vi "Joystick Controls.vi"() -> (3 "Input Cluster":T1)   [LabVIEW 2015]
uses:
  Joytsick/Joytstick Controls Type.ctl
  Global Vars.vi
  <vilib>/Rock Robotics/WPI/Utilities/WPI_GetSetVariantRefNum.vi
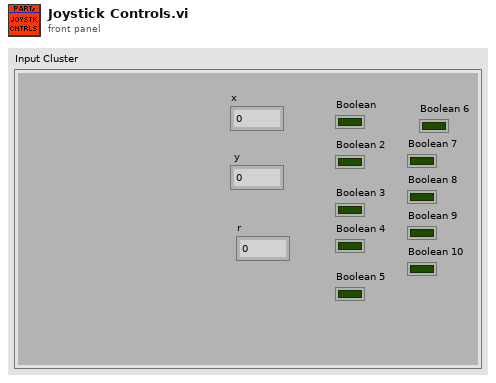
[diagram p1: front panel]
types:
  T1 = typedef "Joytstick Controls Type.ctl" = cluster{"x":dbl, " y":dbl, "r":dbl, "Boolean":bool, "Boolean 2":bool, "Boolean 3":bool, "Boolean 4":bool, "Boolean 5":bool, "Boolean 6":bool, "Boolean 7":bool, "Boolean 8":bool, "Boolean 9":bool, "Boolean 10":bool}
  T2 = typedef "WPI_JoystickDevRef.ctl" = cluster{"Device":T3}
  T3 = typedef "WPI_JoystickDeviceEnum.ctl" = enum16{"USB 0", "USB 1", "USB 2", "USB 3", "USB 4", "USB 5"}
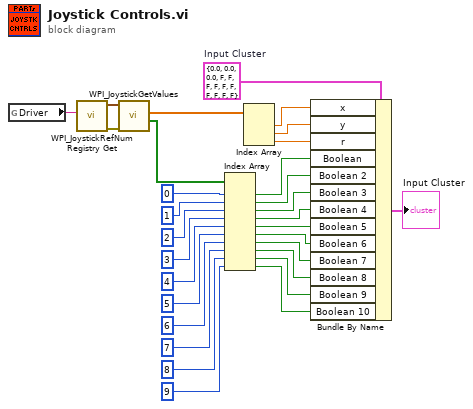
[diagram p0: block diagram]
diagram:
  w18 = T1 {"x"=0.0, " y"=0.0, "r"=0.0, "Boolean"=FALSE, "Boolean 2"=FALSE, "Boolean 3"=FALSE, "Boolean 4"=FALSE, "Boolean 5"=FALSE, "Boolean 6"=FALSE, "Boolean 7"=FALSE, "Boolean 8"=FALSE, "Boolean 9"=FALSE, "Boolean 10"=FALSE}  # Input Cluster
  n1 = global read "Global Vars.vi" "Driver"() -> (w29:string)
  n2 = call <vilib>:"WPI_JoystickRefNum Registry Get.vi"("refnum name"=w29) -> ("error out"=w27:errorcluster, "JoystickDevRef"=w28:T2)  [unwired: 9 in]
  n3 = call <vilib>:"WPI_JoystickGetValues.vi"("error in (no error)"=w27, "JoystickDevRef"=w28) -> ("Buttons"=w26:bool[], "Axes"=w30:dbl[])  [unwired: 5 in, 3 out]
  n4 = Index Array(array=w26, index #1=0 ("index"), index #2=1 ("index"), index #3=2 ("index"), index #4=3 ("index"), index #5=4 ("index"), index #6=5 ("index"), index #7=6 ("index"), index #8=7 ("index"), index #9=8 ("index"), index #10=9 ("index")) -> (element #1=w17:bool, element #2=w16:bool, element #3=w15:bool, element #4=w14:bool, element #5=w13:bool, element #6=w12:bool, element #7=w11:bool, element #8=w10:bool, element #9=w9:bool, element #10=w2:bool)
  n5 = Index Array(array=w30) -> (element #1=w25:dbl, element #2=w24:dbl, element #3=w23:dbl)  [unwired: 3 in]
  n6 = Bundle By Name(cluster=w18, "x"=w25, "y"=w24, "r"=w23, "Boolean"=w17, "Boolean 2"=w16, "Boolean 3"=w15, "Boolean 4"=w14, "Boolean 5"=w13, "Boolean 6"=w12, "Boolean 7"=w11, "Boolean 8"=w10, "Boolean 9"=w9, "Boolean 10"=w2) -> (→"Input Cluster":T1)
